vi "Set DVR.vi"(8 "error in (no error)":errorcluster, 10 "Type Counts":T1, 11 "Local Bus_Int in":refnum<class "Local Bus_Int.lvclass">) -> (0 "error out":errorcluster, 3 "Local Bus_Int out":refnum<class "Local Bus_Int.lvclass">)   [LabVIEW 2021, in "Local Bus_Int.lvclass"]
uses:
  Local Bus_Int.lvclass
  Data Value References.ctl
  <vilib>/TSA/Abstract Data Classes/Abs_Types/Type/Abs_Type.lvclass
  Local Bus.lvclass
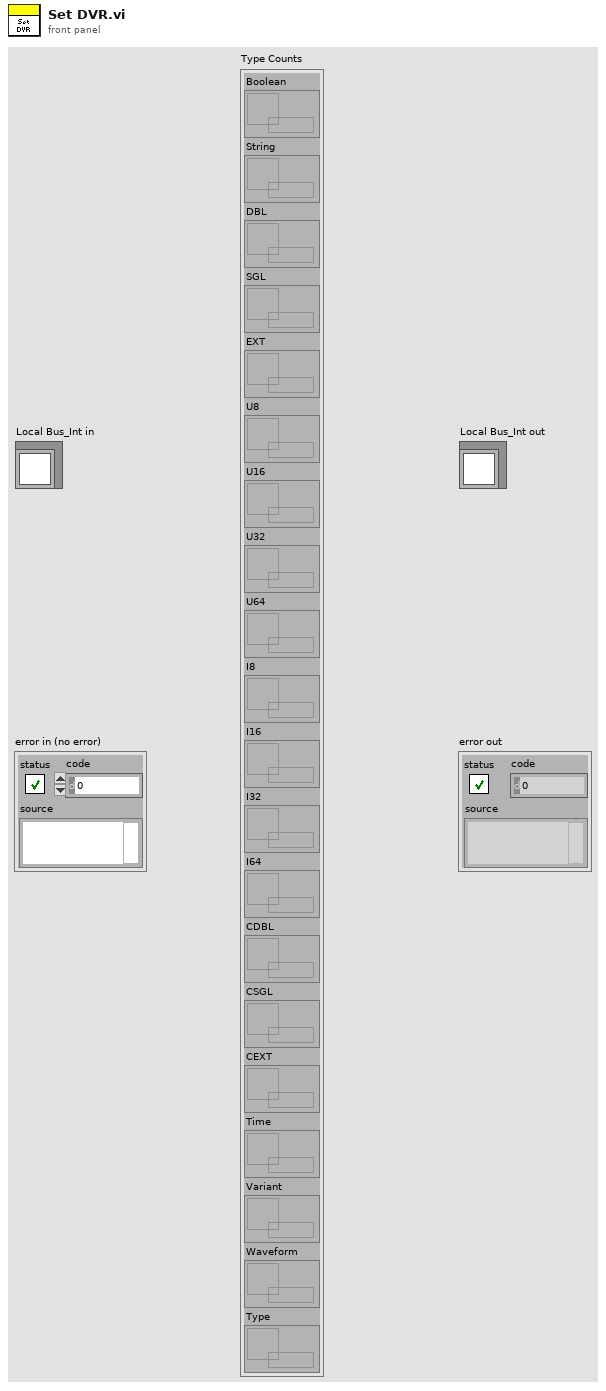
[diagram p1: front panel]
types:
  T1 = typedef "Local Bus.lvclass/Data Value References.ctl" = cluster{"Boolean":refnum<data-value>, "String":refnum<data-value>, "DBL":refnum<data-value>, "SGL":refnum<data-value>, "EXT":refnum<data-value>, "U8":refnum<data-value>, "U16":refnum<data-value>, "U32":refnum<data-value>, "U64":refnum<data-value>, "I8":refnum<data-value>, "I16":refnum<data-value>, "I32":refnum<data-value>, "I64":refnum<data-value>, "CDBL":refnum<data-value>, "CSGL":refnum<data-value>, "CEXT":refnum<data-value>, "Time":refnum<data-value>, "Variant":refnum<data-value>, "Waveform":refnum<data-value>, "Type":refnum<data-value>}
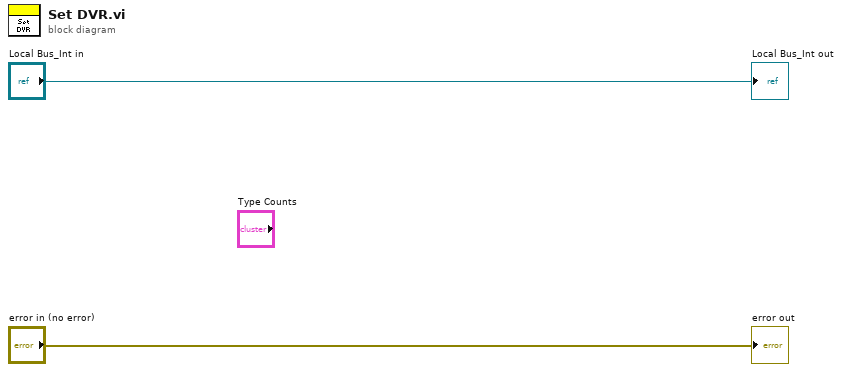
[diagram p0: block diagram]
diagram:
  "error out" <- "error in (no error)"
  "Local Bus_Int out" <- "Local Bus_Int in"
